vi "compute_p_mols.vi"(3 "calibration vol. [ml]":dbl, 4 "humidity [%]":dbl, 5 "pressure [mbar]":dbl, 6 "temperature [°C]":dbl) -> (0 "mols":dbl, 1 "pout":dbl, 2 "wvp":dbl)   [LabVIEW 2015]
doc: "das VI berechnet den Druck (trocken) in der CAL-bottle und die mols im Volumen"
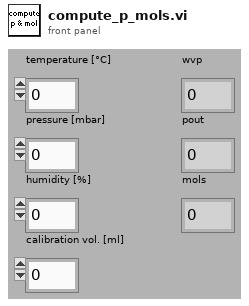
[diagram p1: front panel]
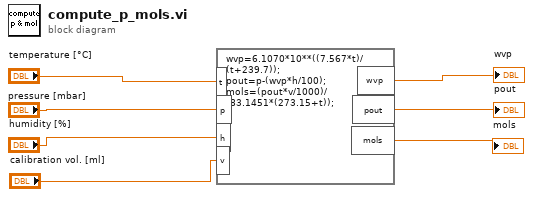
[diagram p0: block diagram]
diagram:
  n1 = formula code="wvp=6.1070*10**((7.567*t)/(t+239.7));\npout=p-(wvp*h/100);\nmols=(pout*v/1000)/(83.1451*(273.15+t));"("t"="temperature [°C]", "p"="pressure [mbar]", "h"="humidity [%]", "v"="calibration vol. [ml]") -> ("wvp"=→"wvp":dbl, "pout"=→"pout":dbl, "mols"=→"mols":dbl)
